vi "PCO_SendBirgerCommand.vi"(7 "inumdelim":i32, 8 "error in (no error)":errorcluster {"code" format="%x"}, 9 "szcmd":string, 11 "hLens":u64) -> (0 "error out":errorcluster {"code" format="%x"}, 1 "strBirger":T1, 2 "ErrorMessage":i32 format="%x", 3 "hLens out":u64)   [LabVIEW 2020, in "SDK.lvlib" / "LensControl.lvlib"]
doc: "<b>Description:</b>\nSends a telegram to a Birger ring device and returns the result in the PCO_Birger structure.\nUsually PCO_GetLensFocus / PCO_SetLensFocus and PCO_GetAperture / PCO_SetAperture are enough. However if you need to send your own command to the Birger ring you can use this function. This is an internally used helper function, which is also exported.\n\n<b>Supported camera type:</b>\npco.edge CLHS, pco.dimax cs\n\n<b>Descriptor dependency:</b>\nNone"
uses:
  LensControl.lvlib
  Structures.lvlib
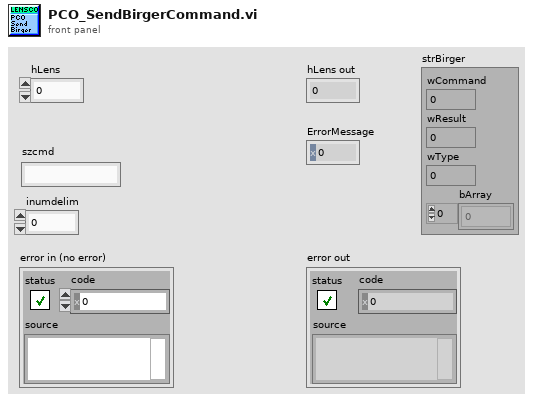
[diagram p1: front panel]
types:
  T1 = cluster{"wCommand":u16, "wResult":u16, "wType":u16, "bArray":u8[]}
  T2 = cluster{"wCommand":u16, "wResult":u16, "wType":u16, "bArray":cluster{u8, u8, u8, u8, u8, u8, u8, u8, u8, u8, u8, u8, u8, u8, u8, u8, u8, u8, u8, u8, u8, u8, u8, u8, u8, u8, u8, u8, u8, u8, u8, u8, u8, u8, u8, u8, u8, u8, u8, u8, u8, u8, u8, u8, u8, u8, u8, u8, u8, u8, u8, u8, u8, u8, u8, u8, u8, u8, u8, u8, u8, u8, u8, u8, u8, u8, u8, u8, u8, u8, u8, u8, u8, u8, u8, u8, u8, u8, u8, u8, u8, u8, u8, u8, u8, u8, u8, u8, u8, u8, u8, u8, u8, u8, u8, u8, u8, u8, u8, u8, u8, u8, u8, u8, u8, u8, u8, u8, u8, u8, u8, u8, u8, u8, u8, u8, u8, u8, u8, u8, u8, u8, u8, u8, u8, u8, u8, u8}}
  T3 = cluster{u8, u8, u8, u8, u8, u8, u8, u8, u8, u8, u8, u8, u8, u8, u8, u8, u8, u8, u8, u8, u8, u8, u8, u8, u8, u8, u8, u8, u8, u8, u8, u8, u8, u8, u8, u8, u8, u8, u8, u8, u8, u8, u8, u8, u8, u8, u8, u8, u8, u8, u8, u8, u8, u8, u8, u8, u8, u8, u8, u8, u8, u8, u8, u8, u8, u8, u8, u8, u8, u8, u8, u8, u8, u8, u8, u8, u8, u8, u8, u8, u8, u8, u8, u8, u8, u8, u8, u8, u8, u8, u8, u8, u8, u8, u8, u8, u8, u8, u8, u8, u8, u8, u8, u8, u8, u8, u8, u8, u8, u8, u8, u8, u8, u8, u8, u8, u8, u8, u8, u8, u8, u8, u8, u8, u8, u8, u8, u8}
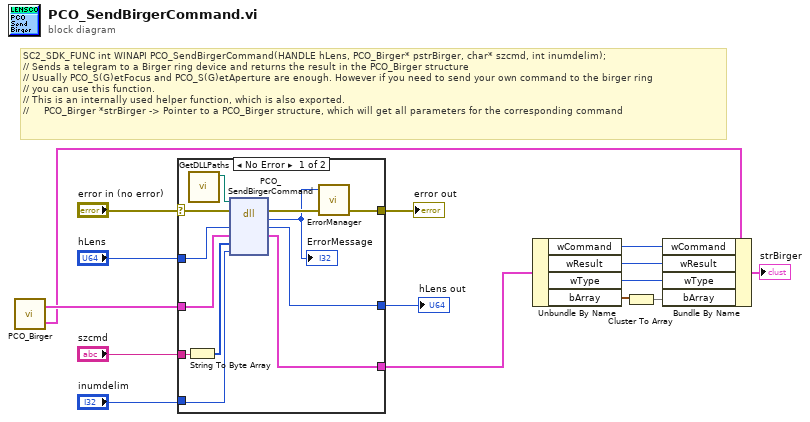
[diagram p0: block diagram]
diagram:
  # "SC2_SDK_FUNC int WINAPI PCO_SendBirgerCommand(HANDLE hLens, PCO_Birger* pstrBirger, char* szcmd, int inumdelim);\n// Sends a telegram to a Birger ring device and returns the result in the PCO_Birger structure\n// Usually PCO_S(G)etFocus and PCO_S(G)etAperture are enough. However if you need to send your own command to the birger ring\n// you can use this function.\n// This is an internally used helper function, which is also exported.\n//     PCO_Birger *strBirger -> Pointer to a PCO_Birger structure, which will get all parameters for the corresponding command"
  n1 = call "PCO_Birger.vi"() -> ("PCO_Birger"=w6:T1, "PCO_Birger_Raw"=w9:T2)  [unwired: 4 in, 2 out]
  n2 = case shown="No Error" "error in (no error)" {
    selector: "error in (no error)" -> [w23 w30]
    tunnel: "hLens" -> [w27 w29]
    tunnel: [w26 w29] -> w14
    tunnel: w9 -> [w25 w28]
    tunnel: "szcmd" -> [w19 _]
    tunnel: "inumdelim" -> [w24 _]
    tunnel: [w22 w30] -> w11
    tunnel: [w17 w28] -> w8
    frame No Error {
      n3 = String To Byte Array(string=w19) -> (unsigned byte array=w18:u8[])
      n4 = call "GetDLLPaths.vi"() -> ("SC2_Cam_Path"=w16:path)  [unwired: 9 in, 2 out]
      n5 = dll-call lib="?" fn="PCO_SendBirgerCommand"(path in=w16, error in=w23, "hLens"=w27, "pstrBirger"=w25, "szcmd"=w18, "inumdelim"=w24) -> (error out=w21:errorcluster, "return type"=w20:i32, "hLens"=w26:u64, "pstrBirger"=w17:T2)  [unwired: 3 in, 1 out]
      "ErrorMessage" <- w20
      n6 = call "ErrorManager.vi"("error in (no error)"=w21, "error code"=w20) -> ("error out"=w22:errorcluster)  [unwired: 3 in]
    }
    frame Error {
    }
  }
  "hLens out" <- w14
  "error out" <- w11
  n7 = Unbundle By Name(w8) -> ("wCommand"=w1:u16, "wResult"=w2:u16, "wType"=w3:u16, "bArray"=w5:T3)
  n8 = Cluster To Array(cluster=w5) -> (array=w4:u8[])
  n9 = Bundle By Name(cluster=w6, "wCommand"=w1, "wResult"=w2, "wType"=w3, "bArray"=w4) -> (→"strBirger":T1)
